vi "Simple UDP - Sender.vi"() -> ()   [LabVIEW 2017]
doc: "The UDP protocol differs from TCP in that there is no error-checking with the packets of information that are sent, and thus no guarantee whatsoever that an intended recipient will actually receive a given piece of data.\n\nUDP does offer the ability to \"broadcast\" data across a network--simply specify an IP Address of all ones (255.255.255.255) to attempt to broadcast information network-wide. Keep in mind that routers and other network hardware will generally refuse to forward the broadcast beyond certain points, so the extent of the broadcast will in practice be limited."
panel:
  out "Array":dbl[](array[numeric])
  in  "Enum":enum16{"RandomNumber", "Text", "Random Array"}(ring)
  in  "data in":string="qqq"
  in  "Stop":bool
  # "Overview: Demonstrates the use of the UDP functions to send data over a UDP connection.\nInstructions:\n1. Run the VI.\n2. Open Simple UDP - Receiver.vi and follow the instructions on its front panel.\n3. Click Stop to stop the VI."
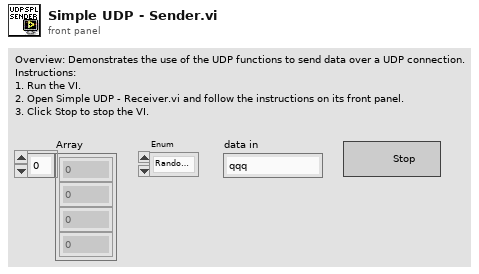
[diagram p1: front panel]
types:
  T1 = enum16{"big-endian, network order", "native, host order", "little-endian"}
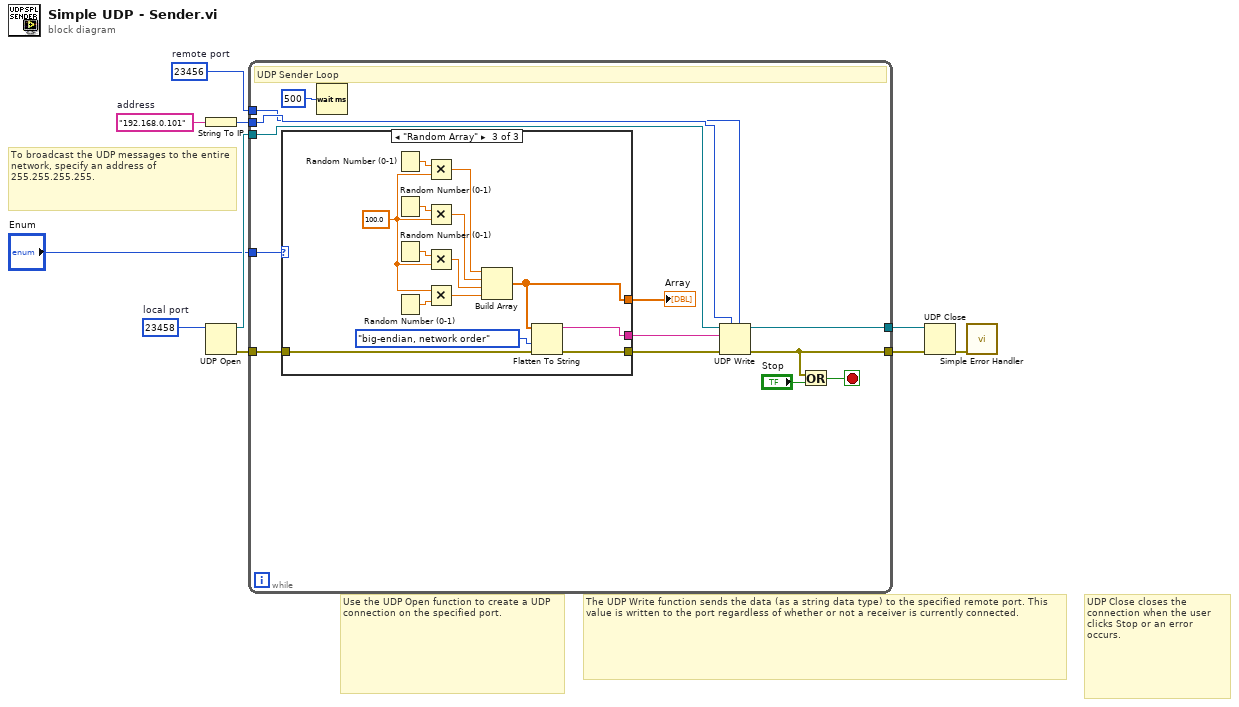
[diagram p0: block diagram]
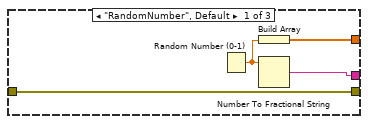
[diagram p2: hidden frame]
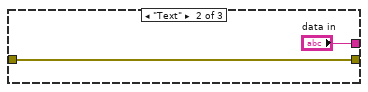
[diagram p3: hidden frame]
diagram:
  w2 = u16 23456  # remote port
  w3 = u16 23458  # local port
  w8 = "192.168.0.101"  # address
  # "To broadcast the UDP messages to the entire network, specify an address of 255.255.255.255."
  # "UDP Close closes the connection when the user clicks Stop or an error occurs."
  # "The UDP Write function sends the data (as a string data type) to the specified remote port. This value is written to the port regardless of whether or not a receiver is currently connected."
  # "Use the UDP Open function to create a UDP connection on the specified port."
  n1 = String To IP(1:w8) -> (0:w6:u32)
  n2 = UDP Open(11:w3) -> (port=w5:refnum<k16>, 0:w4:errorcluster)  [unwired: 4 in, 1 out]
  n3 = while {
    tunnel: [w19] -> w9
    tunnel: w5 -> [w23]
    tunnel: w4 -> [w13]
    tunnel: [w20] -> w10
    tunnel: w6 -> [w18]
    tunnel: w2 -> [w16]
    tunnel: "Enum" -> [w14]
    stop <- w22 stop-if-true
    # "UDP Sender Loop"
    n4 = case shown="\"Random Array\"" w14 {
      tunnel: [w26 "data in" w38] -> w15
      tunnel: w13 -> [w27 w28 w37]
      tunnel: [w27 w28 w36] -> w12
      tunnel: [w24 _ w35] -> w11
      frame "RandomNumber", Default {
        n5 = Random Number (0-1)() -> (number: 0 to 1=w25:dbl)
        n6 = Build Array(w25) -> (w24:dbl[])
        n7 = Number To Fractional String(number=w25) -> (F-format string=w26:string)  [unwired: 3 in]
      }
      frame "Text" {
      }
      frame "Random Array" {
        w30 = 100.0 ("y")
        n8 = Random Number (0-1)() -> (number: 0 to 1=w43:dbl)
        n9 = Random Number (0-1)() -> (number: 0 to 1=w42:dbl)
        n10 = Random Number (0-1)() -> (number: 0 to 1=w41:dbl)
        n11 = Random Number (0-1)() -> (number: 0 to 1=w40:dbl)
        n12 = Multiply(x=w43, y=w30) -> (x*y=w34:dbl)
        n13 = Multiply(x=w42, y=w30) -> (x*y=w33:dbl)
        n14 = Multiply(x=w41, y=w30) -> (x*y=w32:dbl)
        n15 = Multiply(x=w30, y=w40) -> (x*y=w31:dbl)
        n16 = Build Array(w34, w33, w32, w31) -> (w35:dbl[])
        n17 = Flatten To String(anything=w35, byte order (0:big-endian, network order)=T1."big-endian, network order", error in (no error)=w37) -> (data string=w38:string, error out=w36:errorcluster)  [unwired: 1 in, 1 out]
      }
    }
    "Array" <- w11
    n18 = Wait (ms)(milliseconds to wait=u32 500) -> ()  [unwired: 1 out]
    n19 = UDP Write(address=w18, port or service name=w16, connection ID=w23, data in=w15, 8:w12) -> (error out=w19:errorcluster, 3:w20:refnum<k16>)  [unwired: 1 in]
    n20 = Or(x=w19, y="Stop") -> (x .or. y?=w22:bool)
  }
  n21 = UDP Close(connection ID=w10, 8:w9) -> (error out=w7:errorcluster)  [unwired: 1 out]
  n22 = call <vilib>:"Simple Error Handler.vi"("error in (no error)"=w7) -> ()  [unwired: 4 in, 5 out]
